vi "Imbalance Calc.vi"(0 "A":dbl, 1 "B":dbl, 4 "X":dbl) -> (5 "|A-B|>X?":bool)   [LabVIEW 2014]
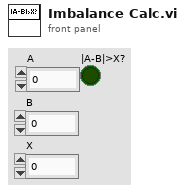
[diagram p1: front panel]
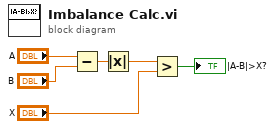
[diagram p0: block diagram]
diagram:
  n1 = Subtract(x="A", y="B") -> (x-y=w4:dbl)
  n2 = Absolute Value(x=w4) -> (abs(x)=w3:dbl)
  n3 = Greater?(x=w3, y="X") -> (0:→"|A-B|>X?":bool)
